vi "GLdrv_FILE_SPACE.vi"(0 "Connection ID":T1, 11 "error in (no error)":errorcluster) -> (4 "Connection ID Out":T1, 6 "Space out":dbl, 15 "error out":errorcluster)   [LabVIEW 2017, in "GL860_Driver.lvlib"]
doc: "CDコマンドで設定されているデバイスの空きスペースの参照\n数値はバイト数を表します。　1234 → 1234Byte\n例) :FILE:SPACE 12345678"
uses:
  GL860_Driver.lvlib
  ConnectionID.ctl
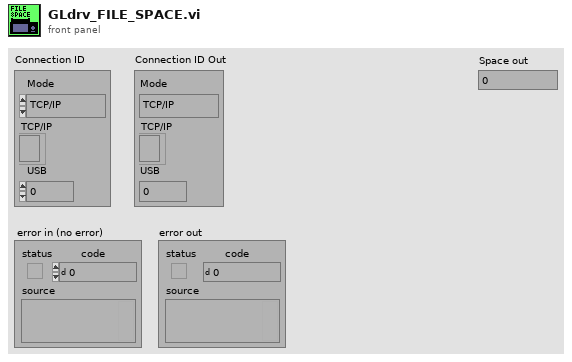
[diagram p1: front panel]
types:
  T1 = typedef "ConnectionID.ctl" = cluster{"Mode":enum16{"TCP/IP", "USB"}, "TCP/IP":refnum<k5>, "USB":i32}
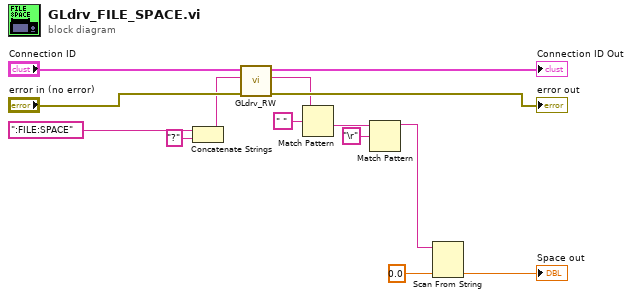
[diagram p0: block diagram]
diagram:
  n1 = Concatenate Strings(":FILE:SPACE" ("Command"), "?" ("string")) -> (w3:string)
  n2 = call "GLdrv_RW.vi"("error in (no error)"="error in (no error)", "data in"=w3, "Connection ID"="Connection ID") -> ("error out"=→"error out":errorcluster, "data out"=w2:string, "Connection ID Out"=→"Connection ID Out":T1)  [unwired: 4 in, 2 out]
  n3 = Match Pattern(string=w2, regular expression=" " ("search string/char (-)")) -> (after substring=w6:string)  [unwired: 4 out]
  n4 = Match Pattern(string=w6, regular expression="\r") -> (before substring=w4:string)  [unwired: 4 out]
  n5 = Scan From String(input string=w4, default 1=0.0 ("Space out")) -> (output 1=→"Space out":dbl)  [unwired: 3 in, 3 out]
